vi "UtilityLib.double 2 string.vi"(2 "Numeric":dbl format="%.8f", 4 "length":u8) -> (16 "String":string, 18 "loss free":bool)   [LabVIEW 2015, in "UtilityLib.lvlib"]
doc: "Tries to do convert a double to a string without loosing digits. The resulting string is supposed to be in a user friendly format."
uses:
  UtilityLib.lvlib
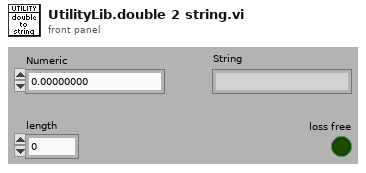
[diagram p1: front panel]
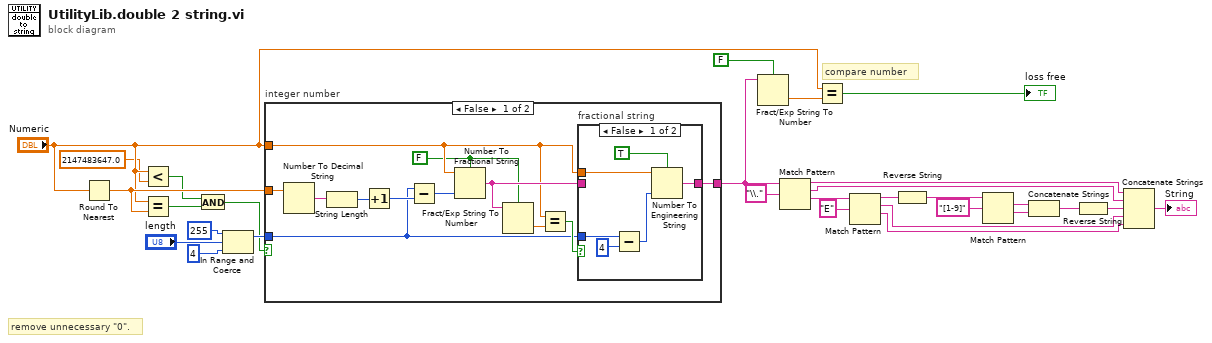
[diagram p0: block diagram]
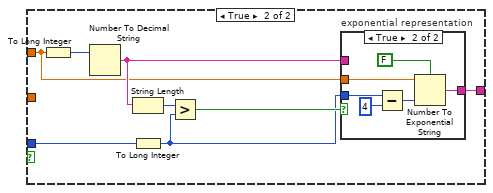
[diagram p3: hidden frame]
diagram:
  # "compare number"
  # "remove unnecessary \"0\"."
  n1 = Round To Nearest(number="Numeric") -> (nearest integer value=w25:dbl)
  n2 = Less?(x="Numeric", y=2147483647.0) -> (x < y?=w2:bool)
  n3 = Equal?(x="Numeric", y=w25) -> (x = y?=w6:bool)
  n4 = And(x=w2, y=w6) -> (x .and. y?=w5:bool)
  n5 = In Range and Coerce(upper limit=u8 255, x="length", lower limit=u8 4) -> (coerced(x)=w28:u8)  [unwired: 1 out]
  n6 = case "integer number" shown="False" w5 {
    tunnel: "Numeric" -> [w31 w51]
    tunnel: w28 -> [w33 w49]
    tunnel: [w32 w50] -> w9
    tunnel: w25 -> [w38 _]
    frame False {
      w30 = FALSE ("use system decimal point (T)")
      n7 = Number To Decimal String(number=w38) -> (decimal integer string=w37:string)  [unwired: 1 in]
      n8 = String Length(string=w37) -> (length=w36:i32)
      n9 = Increment(x=w36) -> (x+1=w35:i32)
      n10 = Subtract(x=w33, y=w35) -> (x-y=w34:i32)
      n11 = Number To Fractional String(use system decimal point (T)=w30, number=w31, precision (6)=w34) -> (F-format string=w39:string)  [unwired: 1 in]
      n12 = Fract/Exp String To Number(use system decimal point (T)=w30, string=w39) -> (number=w41:dbl)  [unwired: 2 in, 1 out]
      n13 = Equal?(x=w31, y=w41) -> (x = y?=w40:bool)
      n14 = case "fractional string" shown="False" w40 {
        tunnel: w31 -> [w47 _]
        tunnel: w39 -> [_ w48]
        tunnel: [w46 w48] -> w32
        tunnel: w33 -> [w44 _]
        frame False {
          n15 = Subtract(x=w44, y=u8 4) -> (x-y=w43:u8)
          n16 = Number To Engineering String(1:TRUE ("use system decimal point (T)"), 2:w43, 4:w47) -> (0:w46:string)  [unwired: 1 in]
        }
        frame True {
        }
      }
    }
    frame True {
      n17 = To Long Integer(number=w51) -> (32bit integer=w56:i32)
      n18 = Number To Decimal String(number=w56) -> (decimal integer string=w52:string)  [unwired: 1 in]
      n19 = String Length(string=w52) -> (length=w55:i32)
      n20 = To Long Integer(number=w49) -> (32bit integer=w53:i32)
      n21 = Greater?(x=w55, y=w53) -> (0:w54:bool)
      n22 = case "exponential representation" shown="True" w54 {
        tunnel: w51 -> [_ w63]
        tunnel: w53 -> [_ w61]
        tunnel: [w57 w62] -> w50
        tunnel: w52 -> [w57 _]
        frame False {
        }
        frame True {
          n23 = Subtract(x=w61, y=4) -> (x-y=w59:i32)
          n24 = Number To Exponential String(number=w63, precision (6)=w59, 1:FALSE ("use system decimal point (T)")) -> (E-format string=w62:string)  [unwired: 1 in]
        }
      }
    }
  }
  n25 = Fract/Exp String To Number(use system decimal point (T)=FALSE, string=w9) -> (number=w8:dbl)  [unwired: 2 in, 1 out]
  n26 = Match Pattern(string=w9, regular expression="\\.") -> (before substring=w24:string, match substring=w23:string, after substring=w12:string)  [unwired: 1 in, 1 out]
  n27 = Equal?(x="Numeric", y=w8) -> (x = y?=→"loss free":bool)
  n28 = Match Pattern(string=w12, regular expression="E") -> (before substring=w14:string, match substring=w20:string, after substring=w21:string)  [unwired: 1 in, 1 out]
  n29 = Reverse String(1:w14) -> (0:w15:string)
  n30 = Match Pattern(string=w15, regular expression="[1-9]") -> (match substring=w17:string, after substring=w18:string)  [unwired: 1 in, 2 out]
  n31 = Concatenate Strings(w17, w18) -> (w19:string)
  n32 = Reverse String(1:w19) -> (0:w22:string)
  n33 = Concatenate Strings(w24, w23, w22, w20, w21) -> (→"String":string)
